vi "get ACS status.vi"(8 "error in (no error)":errorcluster, 11 "Channel in":refnum<class "Channel.lvclass">) -> (0 "error out":errorcluster, 3 "Channel out":refnum<class "Channel.lvclass">)   [LabVIEW 2018, in "Channel.lvclass"]
uses:
  Channel.lvclass
  Channel.lvclass/Channel.ctl
  RxTx/RxTx.lvclass
  Camera/Camera.lvclass
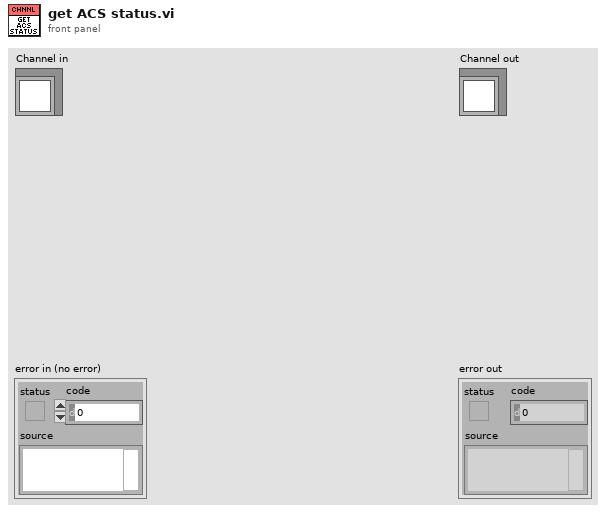
[diagram p1: front panel]
types:
  T1 = cluster{"CCD status":string, "CCD configuration":string, "Acquisition configuration":string, "S4GUI JSON string":string, "WRITE SETUP error":string, "Execution error":string, "SET error":string, "Communication status":string}
  T2 = cluster{"CYCLES_DONE":u16, "LAST_IMAGE_NAME":string, "USED_DISK_SPACE":u16, "FRAMES_DONE":u16, "CCD_STATUS":string, "CURRENT_TEMPERATURE":i16, "TEMPERATURE_STATUS":string, "FRAME_EXPOSURE_TIME":sgl, "ERROR":bool, "SERIAL_NUMBER":u16, "ACQUIRING":bool, "IMAGE_INDEX":u32, "power":bool, "acs mode":bool}
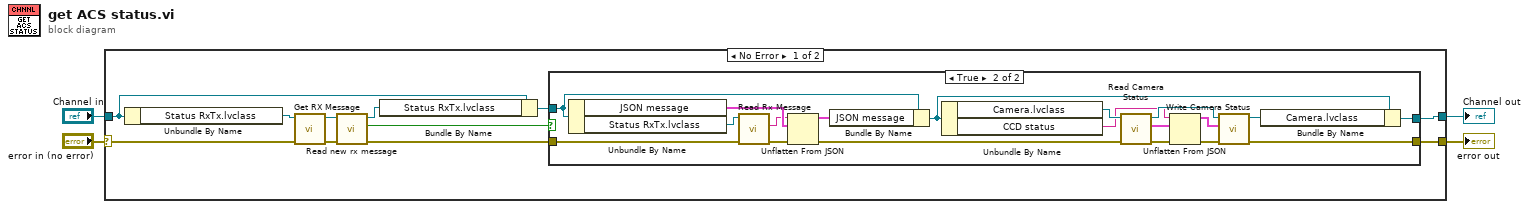
[diagram p0: block diagram]
diagram:
  n1 = case shown="No Error" "error in (no error)" {
    selector: "error in (no error)" -> [w12 w38]
    tunnel: [w15 w38] -> w3
    tunnel: [w14 w37] -> w1
    tunnel: "Channel in" -> [w7 w37]
    frame No Error {
      n2 = Unbundle By Name(w7) -> ("Status RxTx.lvclass"=w13:refnum<class "RxTx.lvclass">)
      n3 = call "Get RX Message.vi"("error in (no error)"=w12, "RxTx in"=w13) -> ("error out"=w11:errorcluster, "RxTx out"=w10:refnum<class "RxTx.lvclass">)  [unwired: 8 in]
      n4 = call-dynamic "Read new rx message.vi"("error in (no error)"=w11, "RxTx in"=w10) -> ("error out"=w8:errorcluster, "new rx message"=w9:bool, "RxTx out"=w6:refnum<class "RxTx.lvclass">)  [unwired: 7 in]
      n5 = Bundle By Name(cluster=w7, "Status RxTx.lvclass"=w6) -> (w5:refnum<class "Channel.lvclass">)
      n6 = case shown="True" w9 {
        tunnel: [w16 w19] -> w15
        tunnel: w5 -> [w17 w29]
        tunnel: [w17 w21] -> w14
        tunnel: w8 -> [w16 w31]
        frame False {
        }
        frame True {
          n7 = Unbundle By Name(w29) -> ("JSON message"=w28:T1, "Status RxTx.lvclass"=w30:refnum<class "RxTx.lvclass">)
          n8 = call "Read Rx Message.vi"("error in (no error)"=w31, "RxTx in"=w30) -> ("error out"=w25:errorcluster, "Rx Message"=w27:string)  [unwired: 7 in, 1 out]
          n9 = Unflatten From JSON(JSON string=w27, type and defaults=w28, error in (no error)=w25) -> (value=w26:T1, error out=w23:errorcluster)  [unwired: 4 in]
          n10 = Bundle By Name(cluster=w29, "JSON message"=w26) -> (w22:refnum<class "Channel.lvclass">)
          n11 = Unbundle By Name(w22) -> ("Camera.lvclass"=w24:refnum<class "Camera.lvclass">, "CCD status"=w20:string)
          n12 = call-dynamic "Read Camera Status.vi"("error in (no error)"=w23, "Camera in"=w24) -> ("error out"=w32:errorcluster, "Camera Status"=w35:T2, "Camera out"=w36:refnum<class "Camera.lvclass">)  [unwired: 7 in]
          n13 = Unflatten From JSON(JSON string=w20, type and defaults=w35, error in (no error)=w32) -> (value=w34:T2, error out=w33:errorcluster)  [unwired: 4 in]
          n14 = call-dynamic "Write Camera Status.vi"("error in (no error)"=w33, "Camera Status"=w34, "Camera in"=w36) -> ("error out"=w19:errorcluster, "Camera out"=w18:refnum<class "Camera.lvclass">)  [unwired: 7 in]
          n15 = Bundle By Name(cluster=w22, "Camera.lvclass"=w18) -> (w21:refnum<class "Channel.lvclass">)
        }
      }
    }
    frame Error {
    }
  }
  "error out" <- w3
  "Channel out" <- w1
